vi "Laundry Data.vi"(0 "File Path In":path, 5 "Input Data 1":string, 7 "Input Data 2":string) -> (4 "File Path Out":path, 8 "output cluster":T1)   [LabVIEW 2014]
uses:
  type defs/ERD_Data.ctl
  <vilib>/Utility/file.llb/Write To Spreadsheet File (string).vi
panel:
  # "UI"
  # "Software Version"
  # "Speed"
  # "Water Level"
  # "Motor Current"
  # "Critical Version"
  # "Non-Critical"
  # "Build & Rev"
  # "Unit Status"
  # "Wet Load Size"
  # "Dry Load Size"
  # "OOB"
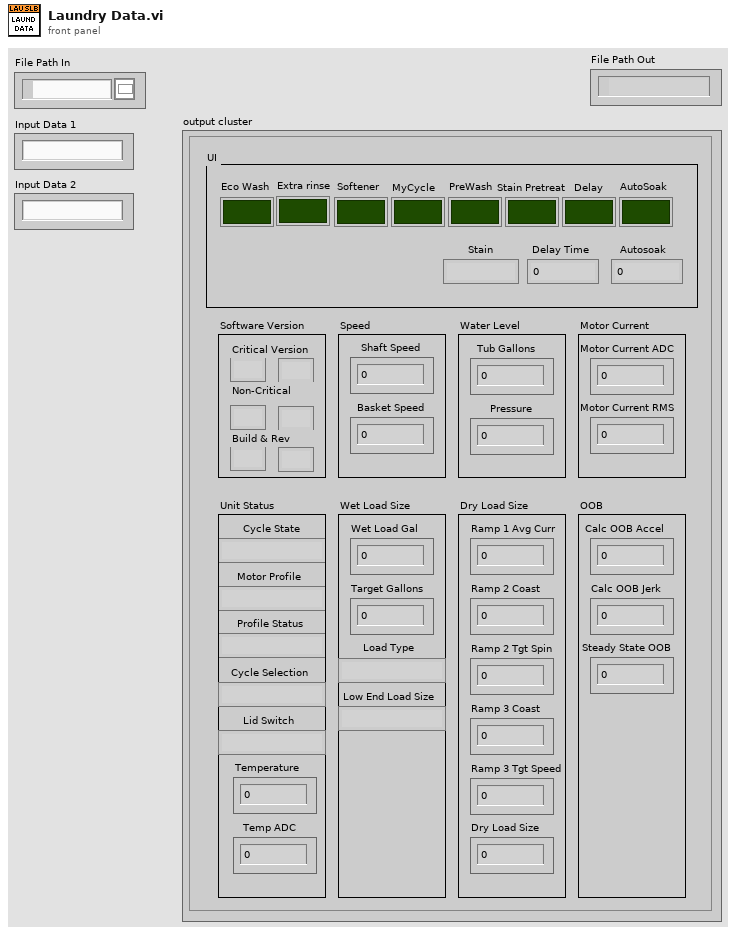
[diagram p1: front panel]
types:
  T1 = typedef "ERD_Data.ctl" = cluster{"Shaft Speed":dbl, "Basket Speed":dbl, "Cycle State":string, "Tub Gallons":dbl, "Pressure":dbl, "Motor Profile":string, "Profile Status":string, "Critical Major":string, "Critical Minor":string, "Non-Critical Minor":string, "Non-Critical Major":string, "Revision":string, "Build":string, "Temperature":dbl, "Motor Current ADC":dbl, "Lid Switch ":string, "Dry Load Size":dbl, "Wet Load Gal":dbl, "Target Gallons":dbl, "Load Type":string, "Cycle Selection":string, "Low End Load Size":string, "Calc OOB Accel":dbl, "Calc OOB Jerk":dbl, "Steady State OOB":dbl, "Eco Wash":bool, "Extra rinse":bool, "Softener":bool, "MyCycle":bool, "PreWash":bool, "Stain Pretreat":bool, "Delay":bool, "AutoSoak":bool, "Stain":string, "Delay Time":dbl, "Autosoak":dbl, "Motor Current RMS":dbl, "Ramp 3 Tgt Speed":dbl, "Ramp 3 Coast":dbl, "Ramp 2 Tgt Spin":dbl, "Ramp 2 Coast":dbl, "Ramp 1 Avg Curr":dbl, "Temp ADC  ":dbl}
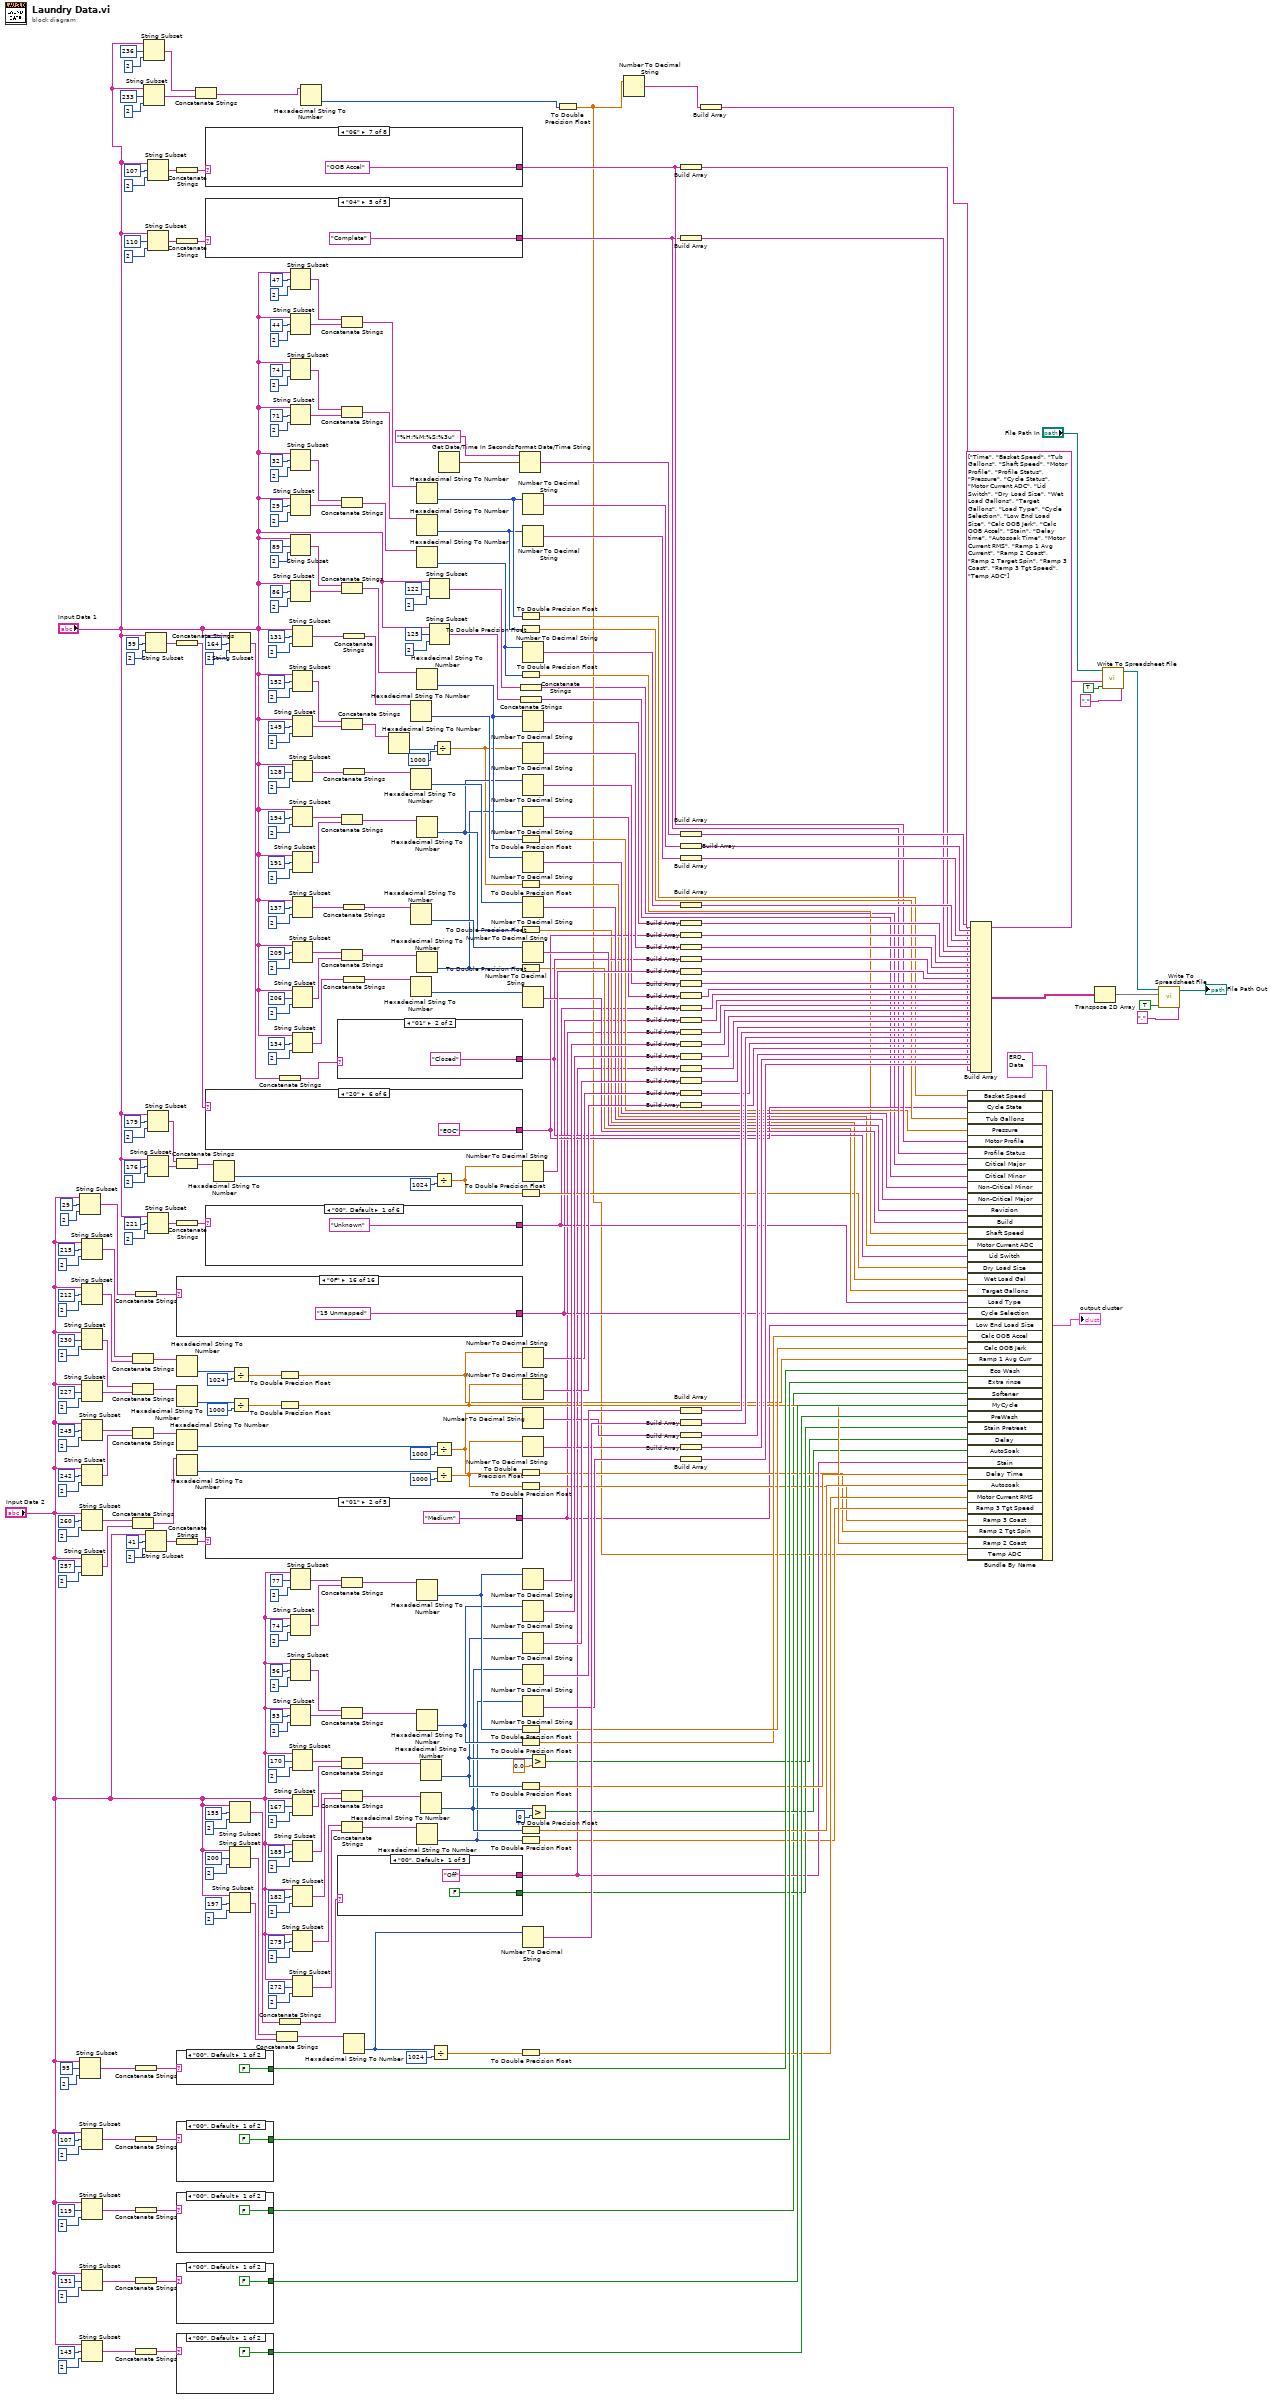
[diagram p0: block diagram]
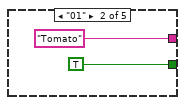
[diagram p2: hidden frame]
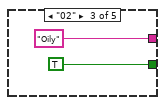
[diagram p3: hidden frame]
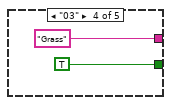
[diagram p4: hidden frame]
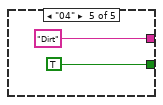
[diagram p5: hidden frame]
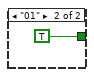
[diagram p6: hidden frame]
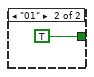
[diagram p7: hidden frame]
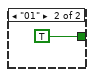
[diagram p8: hidden frame]
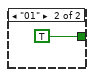
[diagram p9: hidden frame]
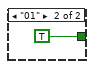
[diagram p10: hidden frame]
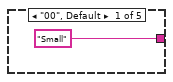
[diagram p11: hidden frame]
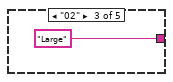
[diagram p12: hidden frame]
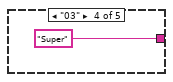
[diagram p13: hidden frame]
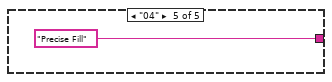
[diagram p14: hidden frame]
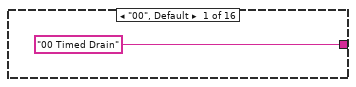
[diagram p15: hidden frame]
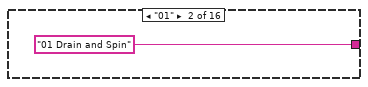
[diagram p16: hidden frame]
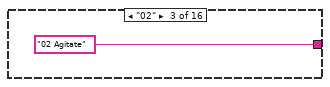
[diagram p17: hidden frame]
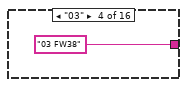
[diagram p18: hidden frame]
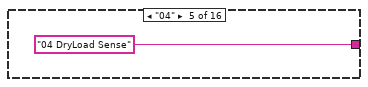
[diagram p19: hidden frame]
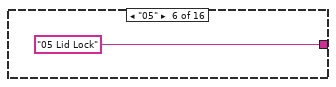
[diagram p20: hidden frame]
diagram:
  n1 = String Subset(string="Input Data 2", offset (0)=29, length (rest)=2 ("length (rest)")) -> (substring=w209:string)
  n2 = String Subset(string="Input Data 2", offset (0)=95, length (rest)=2 ("length (rest)")) -> (substring=w175:string)
  n3 = String Subset(string="Input Data 2", offset (0)=215, length (rest)=2 ("length (rest)")) -> (substring=w116:string)
  n4 = String Subset(string="Input Data 2", offset (0)=212, length (rest)=2 ("length (rest)")) -> (substring=w117:string)
  n5 = String Subset(string="Input Data 2", offset (0)=230, length (rest)=2 ("length (rest)")) -> (substring=w111:string)
  n6 = String Subset(string="Input Data 2", offset (0)=227, length (rest)=2 ("length (rest)")) -> (substring=w110:string)
  n7 = String Subset(string="Input Data 2", offset (0)=245, length (rest)=2 ("length (rest)")) -> (substring=w102:string)
  n8 = String Subset(string="Input Data 2", offset (0)=242, length (rest)=2 ("length (rest)")) -> (substring=w103:string)
  n9 = String Subset(string="Input Data 2", offset (0)=260, length (rest)=2 ("length (rest)")) -> (substring=w97:string)
  n10 = String Subset(string="Input Data 2", offset (0)=257, length (rest)=2 ("length (rest)")) -> (substring=w96:string)
  n11 = String Subset(string="Input Data 2", offset (0)=107, length (rest)=2 ("length (rest)")) -> (substring=w180:string)
  n12 = String Subset(string="Input Data 2", offset (0)=119, length (rest)=2 ("length (rest)")) -> (substring=w172:string)
  n13 = String Subset(string="Input Data 2", offset (0)=131, length (rest)=2 ("length (rest)")) -> (substring=w171:string)
  n14 = String Subset(string="Input Data 2", offset (0)=143, length (rest)=2 ("length (rest)")) -> (substring=w168:string)
  n15 = Concatenate Strings(w116, w117) -> (w118:string)
  n16 = Concatenate Strings(w111, w110) -> (w109:string)
  n17 = Concatenate Strings(w102, w103) -> (w104:string)
  n18 = Concatenate Strings(w97, w96) -> (w95:string)
  n19 = Concatenate Strings(w209) -> (w207:string)
  n20 = Concatenate Strings(w175) -> (w165:string)
  n21 = Concatenate Strings(w180) -> (w164:string)
  n22 = Concatenate Strings(w172) -> (w163:string)
  n23 = Concatenate Strings(w171) -> (w162:string)
  n24 = Concatenate Strings(w168) -> (w143:string)
  n25 = String Subset(string="Input Data 1", offset (0)=236, length (rest)=2 ("length (rest)")) -> (substring=w16:string)
  n26 = String Subset(string="Input Data 1", offset (0)=233, length (rest)=2 ("length (rest)")) -> (substring=w17:string)
  n27 = String Subset(string="Input Data 1", offset (0)=59, length (rest)=2 ("length (rest)")) -> (substring=w307:string)
  n28 = String Subset(string="Input Data 2", offset (0)=41, length (rest)=2 ("length (rest)")) -> (substring=w204:string)
  n29 = String Subset(string="Input Data 1", offset (0)=107, length (rest)=2 ("length (rest)")) -> (substring=w292:string)
  n30 = String Subset(string="Input Data 1", offset (0)=110, length (rest)=2 ("length (rest)")) -> (substring=w297:string)
  n31 = String Subset(string="Input Data 1", offset (0)=179, length (rest)=2 ("length (rest)")) -> (substring=w244:string)
  n32 = String Subset(string="Input Data 1", offset (0)=176, length (rest)=2 ("length (rest)")) -> (substring=w245:string)
  n33 = String Subset(string="Input Data 1", offset (0)=221, length (rest)=2 ("length (rest)")) -> (substring=w213:string)
  n34 = Concatenate Strings(w292) -> (w291:string)
  n35 = Concatenate Strings(w297) -> (w290:string)
  n36 = Concatenate Strings(w307) -> (w319:string)
  n37 = Concatenate Strings(w244, w245) -> (w246:string)
  n38 = Concatenate Strings(w213) -> (w212:string)
  n39 = case shown="\"0F\"" w207 {
    tunnel: ["00 Timed Drain" ("Cycle Selection") "01 Drain and Spin" ("Cycle Selection") "02 Agitate" ("Cycle Selection") "03 FW38" ("Cycle Selection") "04 DryLoad Sense" ("Cycle Selection") "05 Lid Lock" ("Cycle Selection") "06 Volume Fill " ("Cycle Selection") "07 WetLoad Sense " ("Cycle Selection") "08 Load Sense" ("Cycle Selection") "09 OOB Accel" ("Cycle Selection") "10 Unmapped" ("Cycle Selection") "11 Unmapped" ("Cycle Selection") "12 Unmapped" ("Cycle Selection") "13 Unmapped" ("Cycle Selection") "14 Unmapped" ("Cycle Selection") "15 Unmapped" ("Cycle Selection")] -> w43
    frame "00", Default {
    }
    frame "01" {
    }
    frame "02" {
    }
    frame "03" {
    }
    frame "04" {
    }
    frame "05" {
    }
    frame "06" {
    }
    frame "07" {
    }
    frame "08" {
    }
    frame "09" {
    }
    frame "0A" {
    }
    frame "0B" {
    }
    frame "0C" {
    }
    frame "0D" {
    }
    frame "0E" {
    }
    frame "0F" {
    }
  }
  n40 = Hexadecimal String To Number(string=w118) -> (number=w79:u32)  [unwired: 2 in, 1 out]
  n41 = Hexadecimal String To Number(string=w109) -> (number=w85:u32)  [unwired: 2 in, 1 out]
  n42 = Hexadecimal String To Number(string=w104) -> (number=w64:u32)  [unwired: 2 in, 1 out]
  n43 = Hexadecimal String To Number(string=w95) -> (number=w81:u32)  [unwired: 2 in, 1 out]
  n44 = Concatenate Strings(w204) -> (w202:string)
  n45 = case shown="\"00\", Default" w165 {
    tunnel: [FALSE ("Eco Wash") TRUE ("Eco Wash")] -> w41
    frame "00", Default {
    }
    frame "01" {
    }
  }
  n46 = case shown="\"00\", Default" w164 {
    tunnel: [FALSE ("Eco Wash") TRUE ("Eco Wash")] -> w40
    frame "00", Default {
    }
    frame "01" {
    }
  }
  n47 = case shown="\"00\", Default" w163 {
    tunnel: [FALSE ("Eco Wash") TRUE ("Eco Wash")] -> w26
    frame "00", Default {
    }
    frame "01" {
    }
  }
  n48 = case shown="\"00\", Default" w162 {
    tunnel: [FALSE ("Eco Wash") TRUE ("Eco Wash")] -> w42
    frame "00", Default {
    }
    frame "01" {
    }
  }
  n49 = case shown="\"00\", Default" w143 {
    tunnel: [FALSE ("Eco Wash") TRUE ("Eco Wash")] -> w39
    frame "00", Default {
    }
    frame "01" {
    }
  }
  n50 = Concatenate Strings(w16, w17) -> (w11:string)
  n51 = case shown="\"06\"" w291 {
    tunnel: ["Agitate" ("Motor Profile") "Settle" ("Motor Profile") "Jiggle" ("Motor Profile") "Dry load" ("Motor Profile") "Spin Seq" ("Motor Profile") "Fill Spin" ("Motor Profile") "OOB Accel" ("Motor Profile") "Max" ("Motor Profile")] -> w54
    frame "00", Default {
    }
    frame "01" {
    }
    frame "02" {
    }
    frame "03" {
    }
    frame "04" {
    }
    frame "05" {
    }
    frame "06" {
    }
    frame "07" {
    }
  }
  n52 = case shown="\"04\"" w290 {
    tunnel: ["Stop" ("Profile Status") "Active" ("Profile Status") "Pause" ("Profile Status") "Resume" ("Profile Status") "Complete" ("Profile Status")] -> w52
    frame "01", Default {
    }
    frame "00" {
    }
    frame "02" {
    }
    frame "03" {
    }
    frame "04" {
    }
  }
  n53 = case shown="\"20\"" w319 {
    tunnel: ["IDLE" "STANDBY" "DELAY" "RUN" "PAUSE" "EOC"] -> w51
    frame "01", Default {
    }
    frame "02" {
    }
    frame "04" {
    }
    frame "08" {
    }
    frame "10" {
    }
    frame "20" {
    }
  }
  n54 = case shown="\"00\", Default" w212 {
    tunnel: ["Unknown" ("Load Type") "Cotton" ("Load Type") "Synthetic" ("Load Type") "Mixed" ("Load Type") "Low Pressure" ("Load Type") "Leak" ("Load Type")] -> w44
    frame "00", Default {
    }
    frame "01" {
    }
    frame "02" {
    }
    frame "03" {
    }
    frame "04" {
    }
    frame "05" {
    }
  }
  n55 = case shown="\"01\"" w202 {
    tunnel: ["Small" ("Low End Load Size") "Medium" ("Low End Load Size") "Large" ("Low End Load Size") "Super" ("Low End Load Size") "Precise Fill" ("Low End Load Size")] -> w1
    frame "00", Default {
    }
    frame "01" {
    }
    frame "02" {
    }
    frame "03" {
    }
    frame "04" {
    }
  }
  n56 = Hexadecimal String To Number(string=w246) -> (number=w239:u32)  [unwired: 2 in, 1 out]
  n57 = String Subset(string="Input Data 1", offset (0)=164, length (rest)=2 ("length (rest)")) -> (substring=w250:string)
  n58 = String Subset(string="Input Data 2", offset (0)=155, length (rest)=2 ("length (rest)")) -> (substring=w146:string)
  n59 = String Subset(string="Input Data 2", offset (0)=200, length (rest)=2 ("length (rest)")) -> (substring=w129:string)
  n60 = String Subset(string="Input Data 2", offset (0)=197, length (rest)=2 ("length (rest)")) -> (substring=w130:string)
  n61 = Divide(x=w79, y=u32 1024) -> (x/y=w77:dbl)
  n62 = Divide(x=w85, y=u32 1000) -> (x/y=w83:dbl)
  n63 = Concatenate Strings(w129, w130) -> (w131:string)
  n64 = Concatenate Strings(w250) -> (w247:string)
  n65 = To Double Precision Float(number=w77) -> (double precision float=w23:dbl)
  n66 = To Double Precision Float(number=w83) -> (double precision float=w34:dbl)
  n67 = Concatenate Strings(w146) -> (w142:string)
  n68 = String Subset(string="Input Data 1", offset (0)=47, length (rest)=2 ("length (rest)")) -> (substring=w329:string)
  n69 = String Subset(string="Input Data 1", offset (0)=44, length (rest)=2 ("length (rest)")) -> (substring=w328:string)
  n70 = String Subset(string="Input Data 1", offset (0)=74, length (rest)=2 ("length (rest)")) -> (substring=w313:string)
  n71 = String Subset(string="Input Data 1", offset (0)=71, length (rest)=2 ("length (rest)")) -> (substring=w314:string)
  n72 = String Subset(string="Input Data 1", offset (0)=32, length (rest)=2 ("length (rest)")) -> (substring=w334:string)
  n73 = String Subset(string="Input Data 1", offset (0)=29, length (rest)=2 ("length (rest)")) -> (substring=w333:string)
  n74 = String Subset(string="Input Data 1", offset (0)=89, length (rest)=2 ("length (rest)")) -> (substring=w304:string)
  n75 = String Subset(string="Input Data 1", offset (0)=86, length (rest)=2 ("length (rest)")) -> (substring=w305:string)
  n76 = String Subset(string="Input Data 2", offset (0)=77, length (rest)=2 ("length (rest)")) -> (substring=w192:string)
  n77 = String Subset(string="Input Data 2", offset (0)=74, length (rest)=2 ("length (rest)")) -> (substring=w191:string)
  n78 = String Subset(string="Input Data 2", offset (0)=56, length (rest)=2 ("length (rest)")) -> (substring=w199:string)
  n79 = String Subset(string="Input Data 2", offset (0)=53, length (rest)=2 ("length (rest)")) -> (substring=w200:string)
  n80 = String Subset(string="Input Data 1", offset (0)=131, length (rest)=2 ("length (rest)")) -> (substring=w273:string)
  n81 = String Subset(string="Input Data 1", offset (0)=152, length (rest)=2 ("length (rest)")) -> (substring=w260:string)
  n82 = String Subset(string="Input Data 1", offset (0)=149, length (rest)=2 ("length (rest)")) -> (substring=w259:string)
  n83 = String Subset(string="Input Data 1", offset (0)=128, length (rest)=2 ("length (rest)")) -> (substring=w274:string)
  n84 = String Subset(string="Input Data 1", offset (0)=194, length (rest)=2 ("length (rest)")) -> (substring=w224:string)
  n85 = String Subset(string="Input Data 1", offset (0)=191, length (rest)=2 ("length (rest)")) -> (substring=w223:string)
  n86 = String Subset(string="Input Data 1", offset (0)=137, length (rest)=2 ("length (rest)")) -> (substring=w265:string)
  n87 = String Subset(string="Input Data 1", offset (0)=209, length (rest)=2 ("length (rest)")) -> (substring=w233:string)
  n88 = String Subset(string="Input Data 1", offset (0)=206, length (rest)=2 ("length (rest)")) -> (substring=w234:string)
  n89 = String Subset(string="Input Data 1", offset (0)=134, length (rest)=2 ("length (rest)")) -> (substring=w268:string)
  n90 = String Subset(string="Input Data 2", offset (0)=170, length (rest)=2 ("length (rest)")) -> (substring=w156:string)
  n91 = String Subset(string="Input Data 2", offset (0)=167, length (rest)=2 ("length (rest)")) -> (substring=w157:string)
  n92 = String Subset(string="Input Data 2", offset (0)=185, length (rest)=2 ("length (rest)")) -> (substring=w151:string)
  n93 = String Subset(string="Input Data 2", offset (0)=182, length (rest)=2 ("length (rest)")) -> (substring=w150:string)
  n94 = String Subset(string="Input Data 2", offset (0)=275, length (rest)=2 ("length (rest)")) -> (substring=w88:string)
  n95 = String Subset(string="Input Data 2", offset (0)=272, length (rest)=2 ("length (rest)")) -> (substring=w89:string)
  n96 = Hexadecimal String To Number(string=w11) -> (number=w10:u32)  [unwired: 2 in, 1 out]
  n97 = case shown="\"01\"" w247 {
    tunnel: ["Open" ("Lid Switch State") "Closed" ("Lid Switch State")] -> w49
    frame "00", Default {
    }
    frame "01" {
    }
  }
  n98 = case shown="\"00\", Default" w142 {
    tunnel: [FALSE ("Stain Pretreat") TRUE ("Stain Pretreat") TRUE ("Stain Pretreat") TRUE ("Stain Pretreat") TRUE ("Stain Pretreat")] -> w33
    tunnel: ["Off" ("Stain") "Tomato" ("Stain") "Oily" ("Stain") "Grass" ("Stain") "Dirt" ("Stain")] -> w32
    frame "00", Default {
    }
    frame "01" {
    }
    frame "02" {
    }
    frame "03" {
    }
    frame "04" {
    }
  }
  n99 = Concatenate Strings(w329, w328) -> (w327:string)
  n100 = Concatenate Strings(w313, w314) -> (w315:string)
  n101 = Concatenate Strings(w334, w333) -> (w344:string)
  n102 = Concatenate Strings(w304, w305) -> (w302:string)
  n103 = Concatenate Strings(w260, w259) -> (w258:string)
  n104 = Concatenate Strings(w224, w223) -> (w222:string)
  n105 = Concatenate Strings(w233, w234) -> (w235:string)
  n106 = Concatenate Strings(w192, w191) -> (w190:string)
  n107 = Concatenate Strings(w199, w200) -> (w188:string)
  n108 = Concatenate Strings(w156, w157) -> (w158:string)
  n109 = Concatenate Strings(w151, w150) -> (w149:string)
  n110 = Concatenate Strings(w88, w89) -> (w90:string)
  n111 = Concatenate Strings(w273) -> (w271:string)
  n112 = Concatenate Strings(w274) -> (w272:string)
  n113 = Concatenate Strings(w265) -> (w264:string)
  n114 = Concatenate Strings(w268) -> (w267:string)
  n115 = Hexadecimal String To Number(string=w131) -> (number=w123:u32)  [unwired: 2 in, 1 out]
  n116 = Hexadecimal String To Number(string=w258) -> (number=w21:u32)  [unwired: 2 in, 1 out]
  n117 = Hexadecimal String To Number(string=w271) -> (number=w269:u32)  [unwired: 2 in, 1 out]
  n118 = Hexadecimal String To Number(string=w272) -> (number=w270:u32)  [unwired: 2 in, 1 out]
  n119 = Hexadecimal String To Number(string=w264) -> (number=w263:u32)  [unwired: 2 in, 1 out]
  n120 = Hexadecimal String To Number(string=w267) -> (number=w266:u32)  [unwired: 2 in, 1 out]
  n121 = Hexadecimal String To Number(string=w327) -> (number=w323:u32)  [unwired: 2 in, 1 out]
  n122 = Hexadecimal String To Number(string=w315) -> (number=w317:u32)  [unwired: 2 in, 1 out]
  n123 = Hexadecimal String To Number(string=w344) -> (number=w324:u32)  [unwired: 2 in, 1 out]
  n124 = Hexadecimal String To Number(string=w302) -> (number=w306:u32)  [unwired: 2 in, 1 out]
  n125 = Hexadecimal String To Number(string=w222) -> (number=w221:u32)  [unwired: 2 in, 1 out]
  n126 = Hexadecimal String To Number(string=w235) -> (number=w220:u32)  [unwired: 2 in, 1 out]
  n127 = Hexadecimal String To Number(string=w190) -> (number=w189:u32)  [unwired: 2 in, 1 out]
  n128 = Hexadecimal String To Number(string=w188) -> (number=w187:u32)  [unwired: 2 in, 1 out]
  n129 = Hexadecimal String To Number(string=w90) -> (number=w76:u32)  [unwired: 2 in, 1 out]
  n130 = Hexadecimal String To Number(string=w158) -> (number=w137:u32)  [unwired: 2 in, 1 out]
  n131 = Hexadecimal String To Number(string=w149) -> (number=w135:u32)  [unwired: 2 in, 1 out]
  n132 = String Subset(string="Input Data 1", offset (0)=122, length (rest)=2 ("length (rest)")) -> (substring=w279:string)
  n133 = String Subset(string="Input Data 1", offset (0)=125, length (rest)=2 ("length (rest)")) -> (substring=w278:string)
  n134 = Divide(x=w123, y=u32 1024) -> (x/y=w124:dbl)
  n135 = Divide(x=w21, y=u32 1000) -> (x/y=w20:dbl)
  n136 = Divide(x=w239, y=u32 1024) -> (x/y=w62:dbl)
  n137 = Divide(x=w64, y=u32 1000) -> (x/y=w63:dbl)
  n138 = Divide(x=w81, y=u32 1000) -> (x/y=w80:dbl)
  n139 = Get Date/Time In Seconds() -> (seconds since 1Jan1904=w343:timestamp)
  n140 = Format Date/Time String(time format string (%c)="%H:%M:%S:%3u", seconds (now)=w343) -> (date/time string=w338:string)  [unwired: 1 in]
  n141 = To Double Precision Float(number=w323) -> (double precision float=w59:dbl)
  n142 = To Double Precision Float(number=w317) -> (double precision float=w58:dbl)
  n143 = To Double Precision Float(number=w324) -> (double precision float=w22:dbl)
  n144 = Concatenate Strings(w279) -> (w3:string)
  n145 = Concatenate Strings(w278) -> (w25:string)
  n146 = To Double Precision Float(number=w306) -> (double precision float=w50:dbl)
  n147 = To Double Precision Float(number=w20) -> (double precision float=w48:dbl)
  n148 = To Double Precision Float(number=w221) -> (double precision float=w47:dbl)
  n149 = To Double Precision Float(number=w220) -> (double precision float=w46:dbl)
  n150 = To Double Precision Float(number=w62) -> (double precision float=w45:dbl)
  n151 = To Double Precision Float(number=w63) -> (double precision float=w27:dbl)
  n152 = To Double Precision Float(number=w80) -> (double precision float=w28:dbl)
  n153 = To Double Precision Float(number=w189) -> (double precision float=w38:dbl)
  n154 = To Double Precision Float(number=w187) -> (double precision float=w37:dbl)
  n155 = To Double Precision Float(number=w137) -> (double precision float=w36:dbl)
  n156 = To Double Precision Float(number=w135) -> (double precision float=w35:dbl)
  n157 = To Double Precision Float(number=w76) -> (double precision float=w29:dbl)
  n158 = To Double Precision Float(number=w124) -> (double precision float=w30:dbl)
  n159 = Number To Decimal String(number=w323) -> (decimal integer string=w325:string)  [unwired: 1 in]
  n160 = Number To Decimal String(number=w317) -> (decimal integer string=w316:string)  [unwired: 1 in]
  n161 = Number To Decimal String(number=w324) -> (decimal integer string=w339:string)  [unwired: 1 in]
  n162 = Number To Decimal String(number=w306) -> (decimal integer string=w303:string)  [unwired: 1 in]
  n163 = Number To Decimal String(number=w20) -> (decimal integer string=w255:string)  [unwired: 1 in]
  n164 = Number To Decimal String(number=w221) -> (decimal integer string=w219:string)  [unwired: 1 in]
  n165 = Number To Decimal String(number=w220) -> (decimal integer string=w218:string)  [unwired: 1 in]
  n166 = Number To Decimal String(number=w269) -> (decimal integer string=w53:string)  [unwired: 1 in]
  n167 = Number To Decimal String(number=w270) -> (decimal integer string=w55:string)  [unwired: 1 in]
  n168 = Number To Decimal String(number=w263) -> (decimal integer string=w56:string)  [unwired: 1 in]
  n169 = Number To Decimal String(number=w266) -> (decimal integer string=w57:string)  [unwired: 1 in]
  n170 = Number To Decimal String(number=w62) -> (decimal integer string=w237:string)  [unwired: 1 in]
  n171 = Number To Decimal String(number=w23) -> (decimal integer string=w75:string)  [unwired: 1 in]
  n172 = Number To Decimal String(number=w34) -> (decimal integer string=w73:string)  [unwired: 1 in]
  n173 = Number To Decimal String(number=w63) -> (decimal integer string=w72:string)  [unwired: 1 in]
  n174 = Number To Decimal String(number=w80) -> (decimal integer string=w71:string)  [unwired: 1 in]
  n175 = Number To Decimal String(number=w189) -> (decimal integer string=w186:string)  [unwired: 1 in]
  n176 = Number To Decimal String(number=w187) -> (decimal integer string=w185:string)  [unwired: 1 in]
  n177 = Number To Decimal String(number=w137) -> (decimal integer string=w140:string)  [unwired: 1 in]
  n178 = Number To Decimal String(number=w135) -> (decimal integer string=w134:string)  [unwired: 1 in]
  n179 = Number To Decimal String(number=w76) -> (decimal integer string=w70:string)  [unwired: 1 in]
  n180 = Number To Decimal String(number=w123) -> (decimal integer string=w122:string)  [unwired: 1 in]
  n181 = Greater?(x=w137, y=0.0) -> (0:w2:bool)
  n182 = Greater?(x=w135, y=u32 0) -> (0:w31:bool)
  n183 = To Double Precision Float(number=w10) -> (double precision float=w9:dbl)
  n184 = Number To Decimal String(number=w9) -> (decimal integer string=w8:string)  [unwired: 1 in]
  n185 = Build Array(w54) -> (w289:string[])
  n186 = Build Array(w52) -> (w254:string[])
  n187 = Build Array(w338) -> (w337:string[])
  n188 = Build Array(w325) -> (w322:string[])
  n189 = Build Array(w316) -> (w308:string[])
  n190 = Build Array(w339) -> (w318:string[])
  n191 = Build Array(w303) -> (w253:string[])
  n192 = Build Array(w51) -> (w252:string[])
  n193 = Build Array(w255) -> (w251:string[])
  n194 = Build Array(w49) -> (w161:string[])
  n195 = Build Array(w237) -> (w236:string[])
  n196 = Build Array(w219) -> (w217:string[])
  n197 = Build Array(w218) -> (w216:string[])
  n198 = Build Array(w44) -> (w211:string[])
  n199 = Build Array(w43) -> (w206:string[])
  n200 = Build Array(w1) -> (w201:string[])
  n201 = Build Array(w186) -> (w184:string[])
  n202 = Build Array(w185) -> (w183:string[])
  n203 = Build Array(w32) -> (w141:string[])
  n204 = Build Array(w140) -> (w139:string[])
  n205 = Build Array(w75) -> (w74:string[])
  n206 = Build Array(w73) -> (w69:string[])
  n207 = Build Array(w134) -> (w133:string[])
  n208 = Build Array(w122) -> (w121:string[])
  n209 = Build Array(w72) -> (w68:string[])
  n210 = Build Array(w71) -> (w67:string[])
  n211 = Build Array(w70) -> (w66:string[])
  n212 = Build Array(w8) -> (w7:string[])
  n213 = Bundle By Name(cluster=T1 {"Shaft Speed"=0.0, "Basket Speed"=0.0, "Cycle State"="STANDBY", "Tub Gallons"=0.0, "Pressure"=0.0, "Motor Profile"="Agitate", "Profile Status"="Active", "Critical Major"="00", "Critical Minor"="01", "Non-Critical Minor"="32", "Non-Critical Major"="0", "Revision"="0", "Build"="0", "Temperature"=0.0, "Motor Current ADC"=2092.0, "Lid Switch "="Closed", "Dry Load Size"=0.0, "Wet Load Gal"=0.0, "Target Gallons"=0.0, "Load Type"="Unknown", "Cycle Selection"="08 Load Sense", "Low End Load Size"="Small", "Calc OOB Accel"=0.0, "Calc OOB Jerk"=0.0, "Steady State OOB"=0.0, "Eco Wash"=FALSE, "Extra rinse"=FALSE, "Softener"=FALSE, "MyCycle"=FALSE, "PreWash"=FALSE, "Stain Pretreat"=FALSE, "Delay"=FALSE, "AutoSoak"=FALSE, "Stain"="Off", "Delay Time"=0.0, "Autosoak"=0.0, "Motor Current RMS"=0.0, "Ramp 3 Tgt Speed"=0.0, "Ramp 3 Coast"=0.0, "Ramp 2 Tgt Spin"=0.0, "Ramp 2 Coast"=0.0, "Ramp 1 Avg Curr"=0.0, "Temp ADC  "=0.0} ("ERD Data"), "Basket Speed"=w59, "Cycle State"=w51, "Tub Gallons"=w58, "Pressure"=w50, "Motor Profile"=w54, "Profile Status"=w52, "Critical Major"=w3, "Critical Minor"=w25, "Non-Critical Minor"=w53, "Non-Critical Major"=w55, "Revision"=w56, "Build"=w57, "Shaft Speed"=w22, "Motor Current ADC"=w48, "Lid Switch"=w49, "Dry Load Size"=w45, "Wet Load Gal"=w47, "Target Gallons"=w46, "Load Type"=w44, "Cycle Selection"=w43, "Low End Load Size"=w1, "Calc OOB Accel"=w37, "Calc OOB Jerk"=w38, "Ramp 1 Avg Curr"=w23, "Eco Wash"=w41, "Extra rinse"=w40, "Softener"=w26, "MyCycle"=w42, "PreWash"=w39, "Stain Pretreat"=w33, "Delay"=w2, "AutoSoak"=w31, "Stain"=w32, "Delay Time"=w36, "Autosoak"=w35, "Motor Current RMS"=w30, "Ramp 3 Tgt Speed"=w29, "Ramp 3 Coast"=w28, "Ramp 2 Tgt Spin"=w27, "Ramp 2 Coast"=w34, "Temp ADC"=w9) -> (→"output cluster":T1)
  n214 = Build Array(w337, w322, w308, w318, w289, w254, w253, w252, w251, w161, w236, w217, w216, w211, w206, w201, w184, w183, w141, w139, w133, w121, w74, w69, w68, w67, w66, w7) -> (w336:string[][])
  n215 = Transpose 2D Array(2D array=w336) -> (transposed array=w335:string[][])
  n216 = call-poly <vilib>:"Write To Spreadsheet File.vi"("delimiter (\\t)"=",", "append to file? (new file:F)"=TRUE, "1D data"=string[] ["Time", "Basket Speed", "Tub Gallons", "Shaft Speed", "Motor Profile", "Profile Status", "Pressure", "Cycle Status", "Motor Current ADC", "Lid Switch", "Dry Load Size", "Wet Load Gallons", "Target Gallons", "Load Type", "Cycle Selection", "Low End Load Size", "Calc OOB Jerk", "Calc OOB Accel", "Stain", "Delay time", "Autosoak Time", "Motor Current RMS", "Ramp 1 Avg Current", "Ramp 2 Coast", "Ramp 2 Target Spin", "Ramp 3 Coast", "Ramp 3 Tgt Speed", "Temp ADC"], "file path (dialog if empty)"="File Path In") -> ("new file path (Not A Path if cancelled)"=w5:path)  [unwired: 4 in]
  n217 = call-poly <vilib>:"Write To Spreadsheet File.vi"("delimiter (\\t)"=",", "append to file? (new file:F)"=TRUE, "2D data"=w335, "file path (dialog if empty)"=w5) -> ("new file path (Not A Path if cancelled)"=→"File Path Out":path)  [unwired: 4 in]
